vi "Handle Step.vi"(0 "reference in":refnum<class "Stand.lvclass">, 11 "error in (no error)":errorcluster) -> (4 "reference out":refnum<class "Stand.lvclass">, 14 "dt handle step ms":u32, 15 "error out":errorcluster)   [LabVIEW 2019, in "Stand.lvclass"]
uses:
  Stand.lvclass
  Stand.lvclass/Stand.ctl
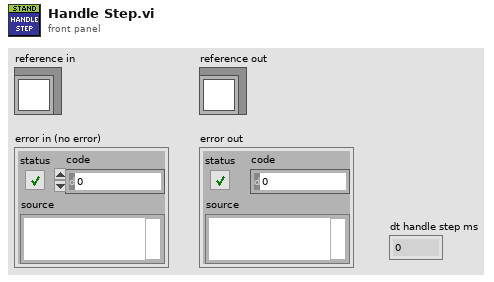
[diagram p1: front panel]
types:
  T1 = typedef "Step_Name.ctl" = enum16{"NONE", "Filling DUT", "Filling Chamber", "Pressure Up DUT", "Abrupt Pressure Release DUT", "Smooth Pressure Release DUT", "Pressure Up Chamber", "Abrupt Pressure Release Chamber", "Smooth Pressure Release Chamber", "Measuring leakage sensor 41.3", "Measuring leakage burette 42", "Low Pressure DUT", "Low Pressure Chamber", "Low Pressure HPP", "ALARM", "Open Air", "MicroStep DUT", "MicroStep CMBR"}
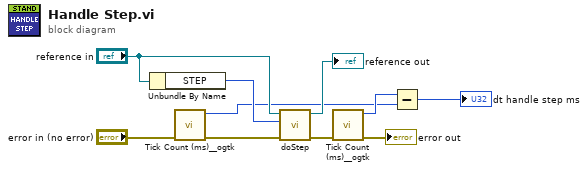
[diagram p0: block diagram]
diagram:
  n1 = Unbundle By Name("reference in") -> ("STEP"=w10:T1)
  n2 = call <userlib>:"Tick Count (ms)__ogtk.vi"("error in (no error)"="error in (no error)") -> ("error out"=w6:errorcluster, "millisecond timer value"=w2:u32)  [unwired: 9 in]
  n3 = call "doStep.vi"("error in (no error)"=w6, "stepName"=w10, "Stand in"="reference in") -> ("error out"=w5:errorcluster, "Stand out"=→"reference out":refnum<class "Stand.lvclass">)  [unwired: 7 in]
  n4 = call <userlib>:"Tick Count (ms)__ogtk.vi"("error in (no error)"=w5) -> ("error out"=→"error out":errorcluster, "millisecond timer value"=w3:u32)  [unwired: 9 in]
  n5 = Subtract(x=w3, y=w2) -> (x-y=→"dt handle step ms":u32)
